vi "XY Graph Get Y Scales Grid Colors.vi"(8 "error in (no error)":errorcluster, 11 "XYGraph in":T1) -> (0 "error out":errorcluster, 1 "Was Tag Found?":bool, 2 "Y Scale.Grid Colors":cluster{"Major Color":u32, "Minor Color":u32}[](array[cluster]), 3 "XYGraph out":T1)   [LabVIEW 2021, in "XY Graph Add-Ons.lvlib"]
uses:
  XY Graph Add-Ons.lvlib
  XY Graph Refnum.ctl
  XY Graph Property Tag List.ctl
  <vilib>/UserTags/UserTags.lvlib
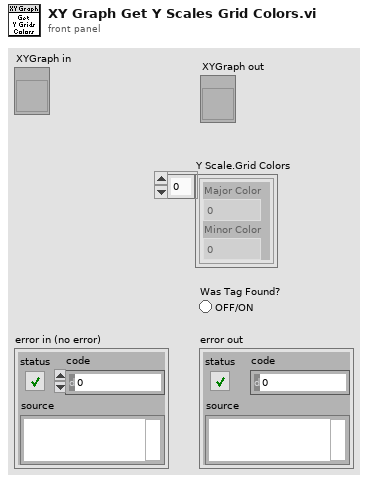
[diagram p1: front panel]
types:
  T1 = typedef "XY Graph Add-Ons.lvlib/XY Graph Refnum.ctl" = refnum<vi>
  T2 = typedef "XY Graph Add-Ons.lvlib/XY Graph Property Tag List.ctl" = enum16{"Max Legend Size", "Preserved Plots", "XScales.GridColors", "YScales.GridColors", "TipStrip String", "TipStrip Visible", "Tool Panels Visibility", "Plots Metadata"}
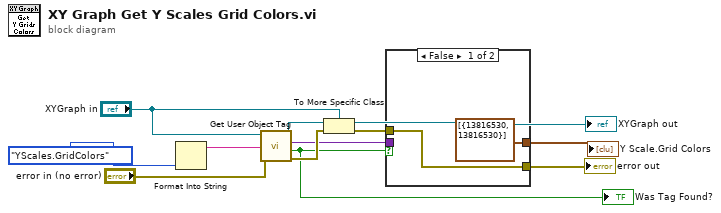
[diagram p0: block diagram]
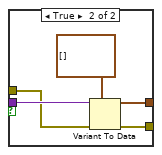
[diagram p2: hidden frame]
diagram:
  n1 = Format Into String(XY_Graph_Property_Tag_List."YScales.GridColors" ("XY Graph Property Tag")) -> (resulting string=w11:string)  [unwired: 3 in, 1 out]
  n2 = call <vilib>:"Get User Object Tag.vi"("error in (no error)"="error in (no error)", "Tag Name"=w11, "Generic Refnum"="XYGraph in") -> ("error out"=w6:errorcluster, "Was Tag Found?"=w5:bool, "Value"=w1:variant, "dup Generic Refnum"=w9:refnum<vi>)  [unwired: 5 in]
  "Was Tag Found?" <- w5
  n3 = To More Specific Class(target class="XYGraph in", reference=w9, error in=w6) -> (specific class reference=→"XYGraph out":T1, error out=w4:errorcluster)
  n4 = case shown="False" w5 {
    tunnel: w1 -> [_ w19]
    tunnel: [cluster{"Major Color":u32, "Minor Color":u32}[] [{"Major Color"=13816530, "Minor Color"=13816530}] ("X Scale.Grid Colors") w17] -> w3
    tunnel: [w13 w16] -> w2
    tunnel: w4 -> [w13 w15]
    frame False {
    }
    frame True {
      n5 = Variant To Data(error in=w15, type=cluster{"Major Color":u32, "Minor Color":u32}[] [] ("X Scale.Grid Colors"), Variant=w19) -> (data=w17:cluster{"Major Color":u32, "Minor Color":u32}[], error out=w16:errorcluster)
    }
  }
  "Y Scale.Grid Colors" <- w3
  "error out" <- w2
